vi "parse_primitive.vi"   [LabVIEW 2018]
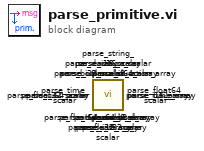
[diagram p0: block diagram]
diagram:
  n1 = call <userlib>:"parse_u64_scalar.vi"() -> ()  [unwired: 5 in, 3 out]
  n2 = call <userlib>:"parse_u64_array.vi"() -> ()  [unwired: 5 in, 3 out]
  n3 = call <userlib>:"parse_u32_scalar.vi"() -> ()  [unwired: 5 in, 3 out]
  n4 = call <userlib>:"parse_u32_array.vi"() -> ()  [unwired: 5 in, 3 out]
  n5 = call <userlib>:"parse_u16_scalar.vi"() -> ()  [unwired: 5 in, 3 out]
  n6 = call <userlib>:"parse_u16_array.vi"() -> ()  [unwired: 5 in, 3 out]
  n7 = call <userlib>:"parse_u8_scalar.vi"() -> ()  [unwired: 5 in, 3 out]
  n8 = call <userlib>:"parse_u8_array.vi"() -> ()  [unwired: 5 in, 3 out]
  n9 = call <userlib>:"parse_time_scalar.vi"() -> ()  [unwired: 5 in, 3 out]
  n10 = call <userlib>:"parse_time_array.vi"() -> ()  [unwired: 5 in, 3 out]
  n11 = call <userlib>:"parse_string_scalar.vi"() -> ()  [unwired: 5 in, 3 out]
  n12 = call <userlib>:"parse_string_array.vi"() -> ()  [unwired: 5 in, 3 out]
  n13 = call <userlib>:"parse_i64_scalar.vi"() -> ()  [unwired: 5 in, 3 out]
  n14 = call <userlib>:"parse_i32_scalar.vi"() -> ()  [unwired: 5 in, 3 out]
  n15 = call <userlib>:"parse_i64_array.vi"() -> ()  [unwired: 5 in, 3 out]
  n16 = call <userlib>:"parse_i32_array.vi"() -> ()  [unwired: 5 in, 3 out]
  n17 = call <userlib>:"parse_i16_scalar.vi"() -> ()  [unwired: 5 in, 3 out]
  n18 = call <userlib>:"parse_i16_array.vi"() -> ()  [unwired: 5 in, 3 out]
  n19 = call <userlib>:"parse_i8_scalar.vi"() -> ()  [unwired: 5 in, 3 out]
  n20 = call <userlib>:"parse_i8_array.vi"() -> ()  [unwired: 5 in, 3 out]
  n21 = call <userlib>:"parse_float64_scalar.vi"() -> ()  [unwired: 5 in, 3 out]
  n22 = call <userlib>:"parse_float64_array.vi"() -> ()  [unwired: 5 in, 3 out]
  n23 = call <userlib>:"parse_float32_scalar.vi"() -> ()  [unwired: 5 in, 3 out]
  n24 = call <userlib>:"parse_float32_array.vi"() -> ()  [unwired: 5 in, 3 out]
  n25 = call <userlib>:"parse_duration_scalar.vi"() -> ()  [unwired: 5 in, 3 out]
  n26 = call <userlib>:"parse_duration_array.vi"() -> ()  [unwired: 5 in, 3 out]
  n27 = call <userlib>:"parse_bool_scalar.vi"() -> ()  [unwired: 5 in, 3 out]
  n28 = call <userlib>:"parse_bool_array.vi"() -> ()  [unwired: 5 in, 3 out]
